vi "WSGI.vi"(8 "error in (no error)":errorcluster, 10 "WSGI Request":T1) -> (0 "error out":errorcluster, 2 "WSGI Response":T1)   [LabVIEW 2021, in "HttpServer.lvlib"]
uses:
  HttpServer.lvlib
  TypeDefs/WSGI.ctl
  TypeDefs/Action.ctl
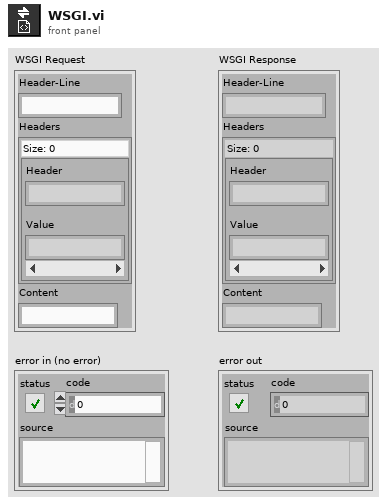
[diagram p1: front panel]
types:
  T1 = typedef "HttpServer.lvlib/WSGI.ctl" = cluster{"Header-Line":string, "Headers":map{string, string}, "Content":string}
  T2 = typedef "HttpServer.lvlib/Action.ctl" = enum8{"noop", "add", "get", "set", "remove"}
  T3 = typedef "HttpServer.lvlib/Request.ctl" = cluster{"Data":string, "Headers":map{string, string}, "Content":string, "Method":string, "Path":string, "Debug":bool, "Query":map{string, string[]}, "Form":map{string, string[]}}
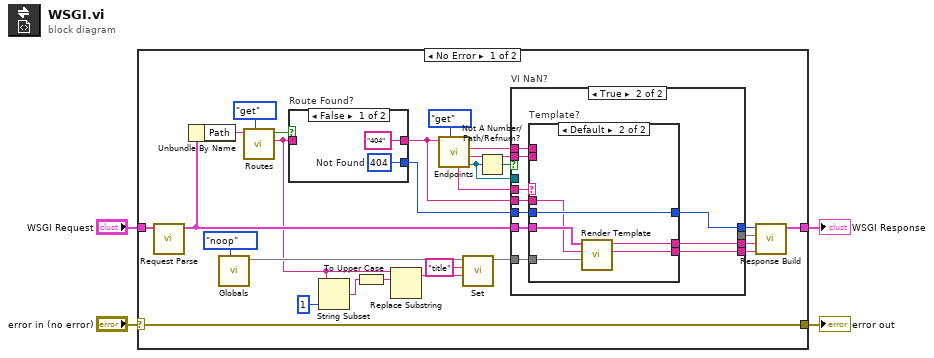
[diagram p0: block diagram]
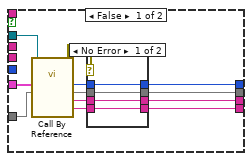
[diagram p2: hidden frame]
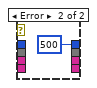
[diagram p3: hidden frame]
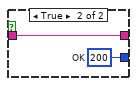
[diagram p5: hidden frame]
diagram:
  n1 = case shown="No Error" "error in (no error)" {
    selector: "error in (no error)" -> [w24 w73]
    tunnel: "WSGI Request" -> [w18 _]
    tunnel: [w26 _] -> w3
    tunnel: [w24 w73] -> w2
    frame No Error {
      n2 = call "Request Parse.vi"("WSGI Request"=w18) -> ("Request"=w17:T3)  [unwired: 10 in]
      n3 = Unbundle By Name(w17) -> ("Path"=w16:string)
      n4 = call "Globals.vi"("Action"=Action."noop") -> ("Globals"=w12:map{string, string[]})  [unwired: 7 in, 3 out]
      n5 = call "Routes.vi"("Action"=Action."get", "Path"=w16) -> ("Endpoint out"=w8:string, "Found?"=w23:bool)  [unwired: 6 in, 2 out]
      n6 = case "Route Found?" shown="False" w23 {
        tunnel: ["404" ("Endpoint out") w72] -> w13
        tunnel: w8 -> [_ w72]
        tunnel: [w69 w71] -> w14
        frame False {
          w69 = 404  # Not Found
        }
        frame True {
          w71 = 200  # OK
        }
      }
      n7 = String Subset(string=w8, length (rest)=1 ("length (rest)")) -> (substring=w6:string)  [unwired: 1 in]
      n8 = To Upper Case(1:w6) -> (0:w5:string)
      n9 = Replace Substring(4:w5, 5:w8) -> (1:w7:string)  [unwired: 2 in, 1 out]
      n10 = call "Endpoints.vi"("Action"=Action."get", "Endpoint"=w13) -> ("VI Refnum out"=w25:refnum<vi>, "Content-Type out"=w20:string, "Content out"=w19:string, "Template out"=w21:string)  [unwired: 4 in, 2 out]
      n11 = call "Set.vi"("Value [Scalar, Cluster, 1D_Clusters, 2D_String]"=w7, "Name"="title", "Variables in"=w12) -> ("Variables out"=w11:map{string, string[]})  [unwired: 7 in, 1 out]
      n12 = Not A Number/Path/Refnum?(number/path/refnum=w25) -> (NaN/Path/Refnum?=w22:bool)
      n13 = case "VI NaN?" shown="True" w22 {
        tunnel: w25 -> [w44 _]
        tunnel: w17 -> [w34 w59]
        tunnel: [w35 w51] -> w30
        tunnel: [w38 _] -> w29
        tunnel: [w39 w57] -> w28
        tunnel: [w42 w56] -> w27
        tunnel: w19 -> [_ w55]
        tunnel: w20 -> [_ w54]
        tunnel: w21 -> [_ w58]
        tunnel: w11 -> [w33 w53]
        tunnel: w14 -> [_ w52]
        tunnel: w13 -> [_ w50]
        frame False {
          n14 = call-by-ref "?"(reference=w44, "Variables in"=w33, "Request"=w34) -> (error out=w43:errorcluster, "Content-Type"=w41:string, "Content"=w40:string, "Headers"=w37:map{string, string}, "Status"=w36:i32)  [unwired: 7 in, 1 out]
          n15 = case shown="No Error" w43 {
            tunnel: [w48 _] -> w42
            tunnel: w41 -> [w48 _]
            tunnel: w40 -> [w47 _]
            tunnel: [w47 _] -> w39
            tunnel: [w46 _] -> w38
            tunnel: w37 -> [w46 _]
            tunnel: w36 -> [w45 _]
            tunnel: [w45 500 ("Status")] -> w35
            frame No Error {
            }
            frame Error {
            }
          }
        }
        frame True {
          n16 = case "Template?" shown="Default" w58 {
            tunnel: w59 -> [_ w66]
            tunnel: [w62 w68] -> w57
            tunnel: [w61 w67] -> w56
            tunnel: w55 -> [w62 _]
            tunnel: w54 -> [w61 _]
            tunnel: w53 -> [_ w65]
            tunnel: w52 -> [w60 w64]
            tunnel: [w60 w64] -> w51
            tunnel: w50 -> [_ w63]
            frame "" {
            }
            frame Default {
              n17 = call "Render Template.vi"("Variables in"=w65, "Endpoint"=w63, "Request"=w66) -> ("Content-Type"=w67:string, "Content out"=w68:string)  [unwired: 7 in]
            }
          }
        }
      }
      n18 = call "Response Build.vi"("Content-Type"=w27, "Content"=w28, "Headers"=w29, "Status"=w30) -> ("WSGI Response"=w26:T1)  [unwired: 7 in]
    }
    frame Error {
    }
  }
  "WSGI Response" <- w3
  "error out" <- w2
